vi "lvstyx_delete_usb_connection.vi"(2 "error in (no error)":errorcluster, 5 "usb conn ptr":u32) -> (0 "error out":errorcluster)   [LabVIEW 2010, in "lib1299.lvlib"]
uses:
  lib1299.lvlib
  cstyx/win32/cstyx.dll
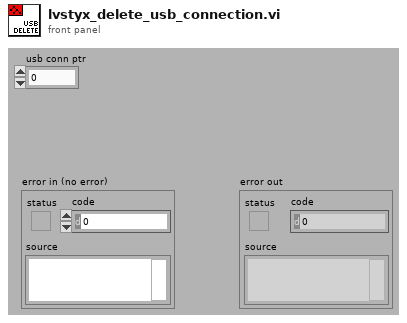
[diagram p1: front panel]
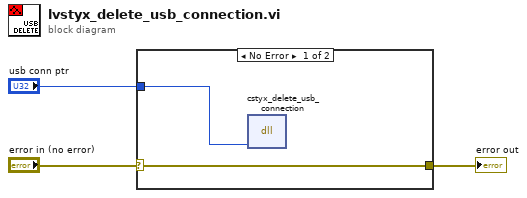
[diagram p0: block diagram]
diagram:
  n1 = case shown="No Error" "error in (no error)" {
    selector: "error in (no error)" -> [w4 w6]
    tunnel: "usb conn ptr" -> [w5 _]
    tunnel: [w4 w6] -> w2
    frame No Error {
      n2 = dll-call lib="C:/work/ads1299evm/lib_1299/Styx/cstyx/win32/cstyx.dll" fn="cstyx_delete_usb_connection"("conn"=w5) -> ()  [unwired: 5 in, 2 out]
    }
    frame Error {
    }
  }
  "error out" <- w2
